vi "Write 1553 Board.vi"(8 "error in (no error)":errorcluster, 10 "1553 Board":refnum<class "1553 Board.lvclass">, 11 "1553 Test in":refnum<class "1553 Test.lvclass">) -> (0 "error out":errorcluster, 3 "1553 Test out":refnum<class "1553 Test.lvclass">)   [LabVIEW 2016, in "1553 Test.lvclass"]
uses:
  1553 Test.lvclass
  1553 Board/1553 Board.lvclass
  1553 Test.lvclass/1553 Test.ctl
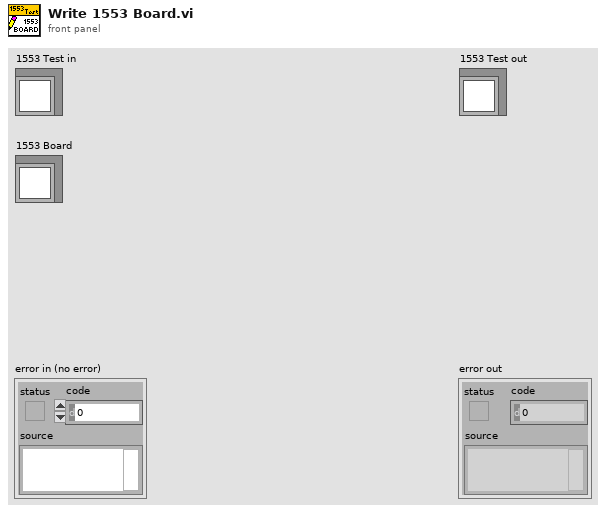
[diagram p1: front panel]
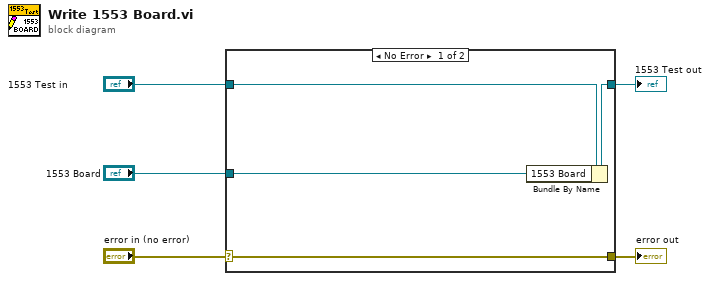
[diagram p0: block diagram]
diagram:
  n1 = case shown="No Error" "error in (no error)" {
    selector: "error in (no error)" -> [w9 w10]
    tunnel: [w9 w10] -> w4
    tunnel: [w7 w11] -> w2
    tunnel: "1553 Test in" -> [w8 w11]
    tunnel: "1553 Board" -> [w6 _]
    frame No Error {
      n2 = Bundle By Name(cluster=w8, "1553 Board"=w6) -> (w7:refnum<class "1553 Test.lvclass">)
    }
    frame Error {
    }
  }
  "error out" <- w4
  "1553 Test out" <- w2
